vi "Server UI Async.vi"(11 "LV Chat Server in":refnum<class "LV Chat Server.lvclass">) -> ()   [LabVIEW 2020, in "LV Chat Server.lvclass"]
uses:
  LV Chat Server.lvclass
panel:
  out "Time Connected":dbl format="%<%H:%M:%S>t"
  out "User IP":string
  out "Users Connected":dbl
  in  "Kick User":bool
  out "Log":string
  in  "Users":i32(listbox)
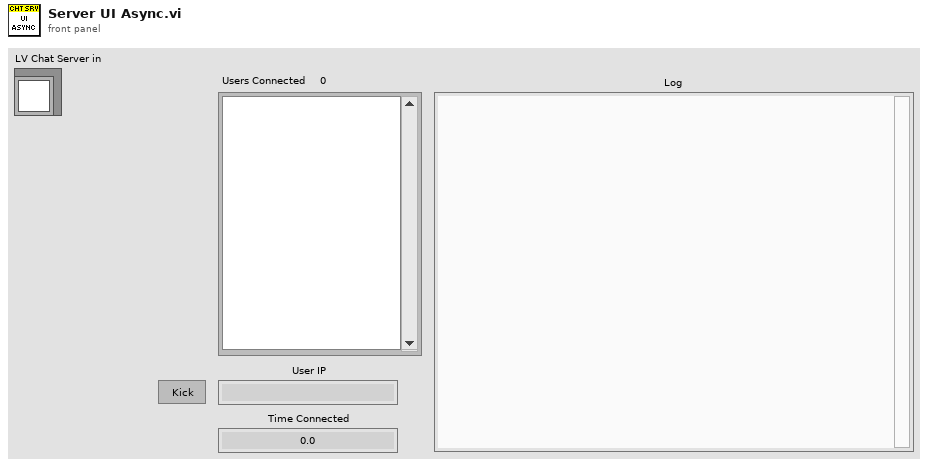
[diagram p1: front panel]
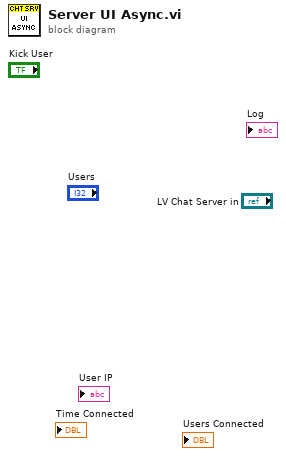
[diagram p0: block diagram]
diagram:
